vi "Get Value for google_protobuf_Syntax.vi"(8 "error in (no error)":errorcluster, 10 "value in LV":u32, 11 "gRPC ID":T1) -> (0 "error out":errorcluster, 2 "value in proto":i32, 3 "gRPC ID Out":T1)   [LabVIEW 2020, in "Measurement Service Client V2.lvlib"]
uses:
  Measurement Service Client V2.lvlib
  <vilib>/gRPC/LabVIEW gRPC Library/Shared/grpcId.ctl
  <vilib>/Utility/error.llb/Error Cluster From Error Code.vi
  <vilib>/Utility/error.llb/Simple Error Handler.vi
  <vilib>/gRPC/LabVIEW gRPC Library/grpc-lvsupport-release.lvlib
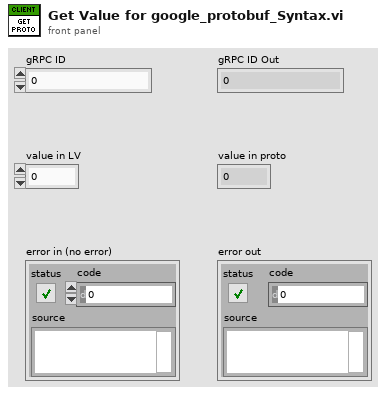
[diagram p1: front panel]
types:
  T1 = typedef "grpc-lvsupport-release.lvlib/grpcId.ctl" = u64
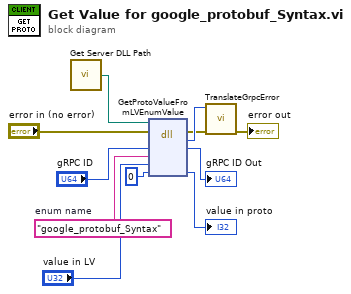
[diagram p0: block diagram]
diagram:
  w8 = "google_protobuf_Syntax"  # enum name
  n1 = call <vilib>:"Get Server DLL Path.vi"() -> ("Server dll path"=w1:path)
  n2 = dll-call lib="?" fn="GetProtoValueFromLVEnumValue"(path in=w1, error in="error in (no error)", "gRPC ID in"="gRPC ID", "enum name"=w8, "value in LV"="value in LV", "value in proto"=0) -> (error out=w3:errorcluster, "error code"=w4:i32, "gRPC ID in"=→"gRPC ID Out":T1, "value in proto"=→"value in proto":i32)  [unwired: 3 in, 1 out]
  n3 = call <vilib>:"TranslateGrpcError.vi"("error in"=w3, "Error Code"=w4) -> ("error out"=→"error out":errorcluster)  [unwired: 9 in]
